vi "Windows Simulate Resolver.vi"() -> ()   [LabVIEW 2010]
panel:
  in  "Scaling Factor 2":fxp<+/-,19,5>
  out "Resolver":dynamicdata(graph)
  in  "Position (deg)":dbl(slide) caption="Position" scale=0.0..360.0 scale format="%.2f"
  in  "stop":bool
  in  "Scaling Factor":fxp<+/-,19,5>
  # "Run-Time"
  # "Display"
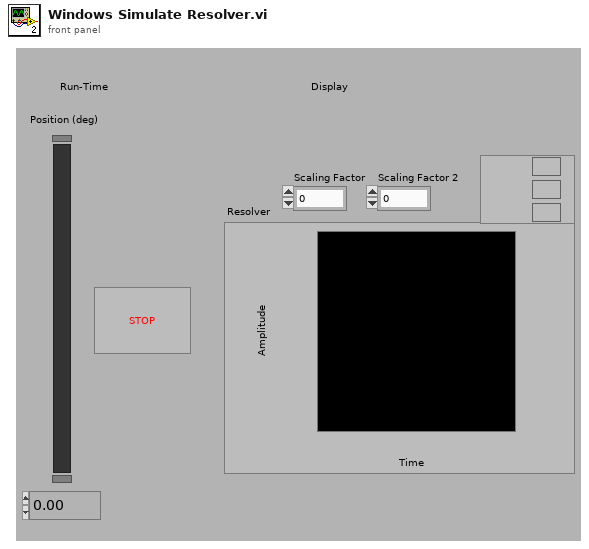
[diagram p1: front panel]
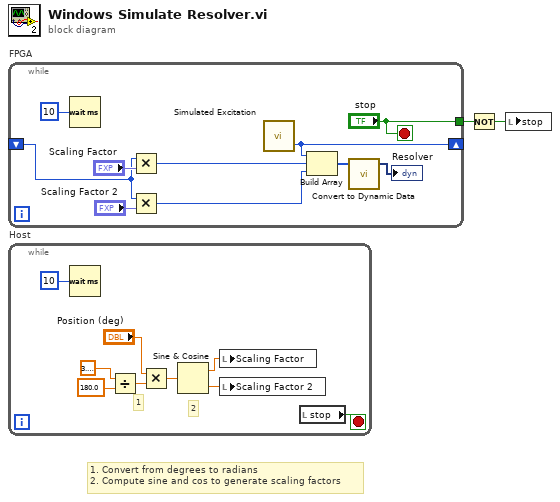
[diagram p0: block diagram]
diagram:
  # "1. Convert from degrees to radians\n2. Compute sine and cos to generate scaling factors"
  n1 = while "FPGA" {
    shift-right: [w6] -> _
    shift-left: _ -> [w3]
    tunnel: ["stop"] -> w2
    stop <- "stop" stop-if-true
    n2 = Wait (ms)(milliseconds to wait=u32 10) -> ()  [unwired: 1 out]
    n3 = Multiply(x=w3, y="Scaling Factor") -> (x*y=w5:i16)
    n4 = Multiply(x=w3, y="Scaling Factor 2") -> (x*y=w4:i16)
    n5 = call "Simulated Excitation.vi"() -> ("Analog Input"=w6:i16)  [unwired: 3 in]
    n6 = Build Array(w6, w5, w4) -> (w11:i16[])
    n7 = call "Convert to Dynamic Data"("Array"=w11) -> ("Dynamic Data Type"=→"Resolver":dynamicdata)  [unwired: 3 in]
  }
  n8 = while "Host" {
    stop <- w21 stop-if-true
    # "2"
    # "1"
    n9 = Wait (ms)(milliseconds to wait=u32 10) -> ()  [unwired: 1 out]
    n10 = Divide(x=3.141592653589793, y=180.0) -> (x/y=w15:dbl)
    n11 = Multiply(x="Position (deg)", y=w15) -> (x*y=w13:dbl)
    n12 = Sine & Cosine(0:w13) -> (1:w19:dbl, 2:w18:dbl)
    n13 = local write "Scaling Factor"(w19) -> ()
    n14 = local write "Scaling Factor 2"(w18) -> ()
    n15 = local read "stop"() -> (w21:bool)
  }
  n16 = Not(x=w2) -> (.not. x?=w1:bool)
  n17 = local write "stop"(w1) -> ()
